vi "Lesson 3 - Exercise 3.1.1 - Complex Relationship Equations.vi"() -> ()   [LabVIEW 2016]
uses:
  <vilib>/Analysis/NI_AALBase.lvlib
panel:
  in  "Phase, deg":i32=30 step=15
  in  "Amplitude":i32=6 step=15
  out "A*Cos(f+phase)":dbl[](graph)=[5.196152422706632, 4.997527444260597, 4.779179508145178, 4.541970333910539, 4.286836077796821, 4.01478363815315, 3.7268866816698627, 3.4242814061065916, 3.1081620562387817, 2.779776210719172, 2.440419858454802, 2.091432283930893, 1.7341907816668303, 1.3701052206639366, 1.0006124802966145, 0.627170779605923, 0.25125392237519883, -0.12565451930013938, -0.5020670599938918, -0.8764981713744672, -1.2474701449065546, -1.6135189236915917, -1.973199880431498, -2.3250935187126154, -2.6678110751095634, -2.9999999999999973, -3.320349295460063, -3.6275946891742468, -3.920523623940631, -4.19798004308019, -4.458868952864364, -4.702160743955037, -4.926895254802223, -5.1321855609630385, -5.317221475387287, -5.4812727458556045, -5.623691936951348, -5.743916985192403, -5.84147341723896, -5.915976222423029, -5.967131372209639, -5.99473698059315, -5.998684100849072, -5.978957155497026, -5.93563399777793, -5.868885604402834, -5.778975400785949, -5.666258221424887, -5.531178909531004, -5.374270561436479, -5.196152422706633, -4.997527444260599, -4.779179508145179, -4.541970333910541, -4.286836077796822, -4.014783638153152, -3.7268866816698645, -3.4242814061065934, -3.1081620562387835, -2.7797762107191737, -2.4404198584548036, -2.091432283930895, -1.734190781666832, -1.3701052206639384, -1.0006124802966163, -0.6271707796059248, -0.2512539223752006, 0.1256545193001377, 0.50206705999389, 0.8764981713744657, 1.247470144906553, 1.6135189236915903, 1.9731998804314965, 2.325093518712614, 2.667811075109562, 2.9999999999999964, 3.320349295460062, 3.627594689174246, 3.92052362394063, 4.1979800430801895, 4.458868952864363, 4.702160743955036, 4.926895254802222, 5.132185560963038, 5.317221475387287, 5.481272745855604, 5.623691936951348, 5.743916985192403, 5.84147341723896, 5.915976222423029, 5.967131372209639, 5.99473698059315, 5.998684100849073, 5.978957155497027, 5.935633997777931, 5.868885604402836, 5.77897540078595, 5.666258221424889, 5.531178909531005, 5.3742705614364805]
  in  "I":dbl=5.196152422706632 format="%#.2g"
  in  "Q":dbl=2.9999999999999996 format="%#.2g"
  in  "stop":bool
  out "Q * Sin(f)":dbl[](graph)=[0.0, 0.18837155858794008, 0.3759997006929127, 0.5621439437571738, 0.7460696614945643, 0.9270509831248421, 1.1043736580540338, 1.2773378746952178, 1.4452610223051456, 1.6074803849369896, 1.7633557568774192, 1.9122719692460688, 2.0536413177860657, 2.186905882264234, 2.3115397283273675, 2.4270509831248415, 2.532983776506045, 2.62892004013159, 2.7144811573980583, 2.7893294576647536, 2.8531695488854605, 2.905749483385893, 2.9468617521860656, 2.976344103943433, 2.9940801852848145, 2.9999999999999996, 2.9940801852848145, 2.976344103943433, 2.9468617521860656, 2.905749483385893, 2.8531695488854605, 2.7893294576647536, 2.7144811573980583, 2.62892004013159, 2.532983776506045, 2.4270509831248415, 2.3115397283273675, 2.186905882264234, 2.0536413177860657, 1.9122719692460686, 1.7633557568774192, 1.6074803849369894, 1.4452610223051456, 1.2773378746952175, 1.1043736580540338, 0.9270509831248419, 0.7460696614945643, 0.5621439437571736, 0.3759997006929128, 0.18837155858793986, 5.551115123125783e-17, -0.1883715585879403, -0.37599970069291266, -0.562143943757174, -0.7460696614945642, -0.9270509831248424, -1.1043736580540338, -1.277337874695218, -1.4452610223051456, -1.6074803849369899, -1.7633557568774192, -1.912271969246069, -2.0536413177860657, -2.1869058822642344, -2.3115397283273675, -2.427050983124842, -2.532983776506045, -2.6289200401315904, -2.7144811573980583, -2.7893294576647536, -2.8531695488854605, -2.905749483385893, -2.9468617521860656, -2.976344103943433, -2.9940801852848145, -2.9999999999999996, -2.9940801852848145, -2.976344103943433, -2.9468617521860656, -2.905749483385893, -2.8531695488854605, -2.7893294576647536, -2.7144811573980583, -2.62892004013159, -2.532983776506045, -2.4270509831248415, -2.3115397283273675, -2.186905882264234, -2.0536413177860657, -1.9122719692460686, -1.7633557568774192, -1.6074803849369894, -1.4452610223051456, -1.2773378746952175, -1.1043736580540338, -0.9270509831248419, -0.7460696614945643, -0.5621439437571736, -0.3759997006929128, -0.18837155858793986]
  out "I * Cos(f)":dbl[](graph)=[5.196152422706632, 5.185899002848537, 5.15517920883809, 5.104114277667713, 5.032905739291384, 4.941834621277992, 4.831260339723896, 4.7016192808018085, 4.5534230785439265, 4.387256595656161, 4.20377561533222, 4.003704253176961, 3.787832099452895, 3.5570111029281697, 3.312152208623981, 3.054221762730764, 2.7842376988812427, 2.50326552083145, 2.2124140974041655, 1.9128312862902854, 1.6056994039789045, 1.2922305596943, 0.9736618717545665, 0.6512505852308165, 0.32626911017524973, 7.771561172376096e-16, -0.32626911017524984, -0.6512505852308149, -0.9736618717545666, -1.2922305596942985, -1.6056994039789045, -1.9128312862902839, -2.2124140974041655, -2.5032655208314485, -2.7842376988812427, -3.0542217627307626, -3.312152208623981, -3.5570111029281684, -3.787832099452895, -4.00370425317696, -4.20377561533222, -4.38725659565616, -4.5534230785439265, -4.701619280801808, -4.831260339723896, -4.941834621277991, -5.032905739291384, -5.104114277667712, -5.15517920883809, -5.1858990028485366, -5.196152422706632, -5.1858990028485366, -5.15517920883809, -5.104114277667712, -5.032905739291384, -4.941834621277991, -4.831260339723896, -4.701619280801808, -4.5534230785439265, -4.38725659565616, -4.20377561533222, -4.00370425317696, -3.787832099452895, -3.5570111029281692, -3.312152208623981, -3.0542217627307635, -2.7842376988812427, -2.50326552083145, -2.2124140974041655, -1.9128312862902854, -1.6056994039789045, -1.2922305596943002, -0.9736618717545665, -0.6512505852308169, -0.32626911017524973, -1.4432899320127035e-15, 0.32626911017524984, 0.651250585230814, 0.9736618717545666, 1.2922305596942973, 1.6056994039789045, 1.9128312862902825, 2.2124140974041655, 2.5032655208314467, 2.7842376988812427, 3.0542217627307604, 3.312152208623981, 3.557011102928166, 3.787832099452895, 4.0037042531769576, 4.20377561533222, 4.387256595656157, 4.5534230785439265, 4.701619280801805, 4.831260339723896, 4.941834621277988, 5.032905739291384, 5.104114277667709, 5.15517920883809, 5.185899002848534]
  out "I*Cos(f) - Q*Sin(f)":dbl[](graph)=[5.196152422706632, 4.997527444260597, 4.779179508145178, 4.541970333910539, 4.28683607779682, 4.014783638153149, 3.726886681669862, 3.4242814061065907, 3.108162056238781, 2.779776210719171, 2.440419858454801, 2.0914322839308923, 1.7341907816668294, 1.3701052206639357, 1.0006124802966134, 0.6271707796059225, 0.2512539223751977, -0.12565451930014016, -0.5020670599938928, -0.8764981713744682, -1.247470144906556, -1.6135189236915928, -1.973199880431499, -2.3250935187126167, -2.6678110751095647, -2.9999999999999987, -3.320349295460064, -3.627594689174248, -3.9205236239406323, -4.197980043080191, -4.458868952864365, -4.702160743955037, -4.926895254802224, -5.1321855609630385, -5.317221475387288, -5.481272745855604, -5.6236919369513485, -5.743916985192403, -5.84147341723896, -5.915976222423029, -5.967131372209639, -5.994736980593149, -5.998684100849072, -5.978957155497025, -5.935633997777929, -5.868885604402832, -5.778975400785948, -5.6662582214248856, -5.531178909531003, -5.374270561436476, -5.196152422706632, -4.997527444260596, -4.779179508145178, -4.5419703339105375, -4.28683607779682, -4.0147836381531485, -3.726886681669862, -3.42428140610659, -3.108162056238781, -2.77977621071917, -2.440419858454801, -2.0914322839308914, -1.7341907816668294, -1.3701052206639348, -1.0006124802966134, -0.6271707796059216, -0.2512539223751977, 0.1256545193001406, 0.5020670599938928, 0.8764981713744682, 1.247470144906556, 1.6135189236915926, 1.973199880431499, 2.3250935187126163, 2.6678110751095647, 2.9999999999999982, 3.320349295460064, 3.627594689174247, 3.9205236239406323, 4.19798004308019, 4.458868952864365, 4.702160743955036, 4.926895254802224, 5.132185560963037, 5.317221475387288, 5.481272745855602, 5.6236919369513485, 5.7439169851924, 5.84147341723896, 5.915976222423026, 5.967131372209639, 5.994736980593147, 5.998684100849072, 5.978957155497023, 5.935633997777929, 5.868885604402831, 5.778975400785948, 5.666258221424883, 5.531178909531003, 5.374270561436473]
  # "Run the program.\nCreate a signal by controlling the Phase (at the top).\nNotice how the amplitudes of two individual signals below are manipulated such that when combined, they also create the original signal."
  # "How does this work?"
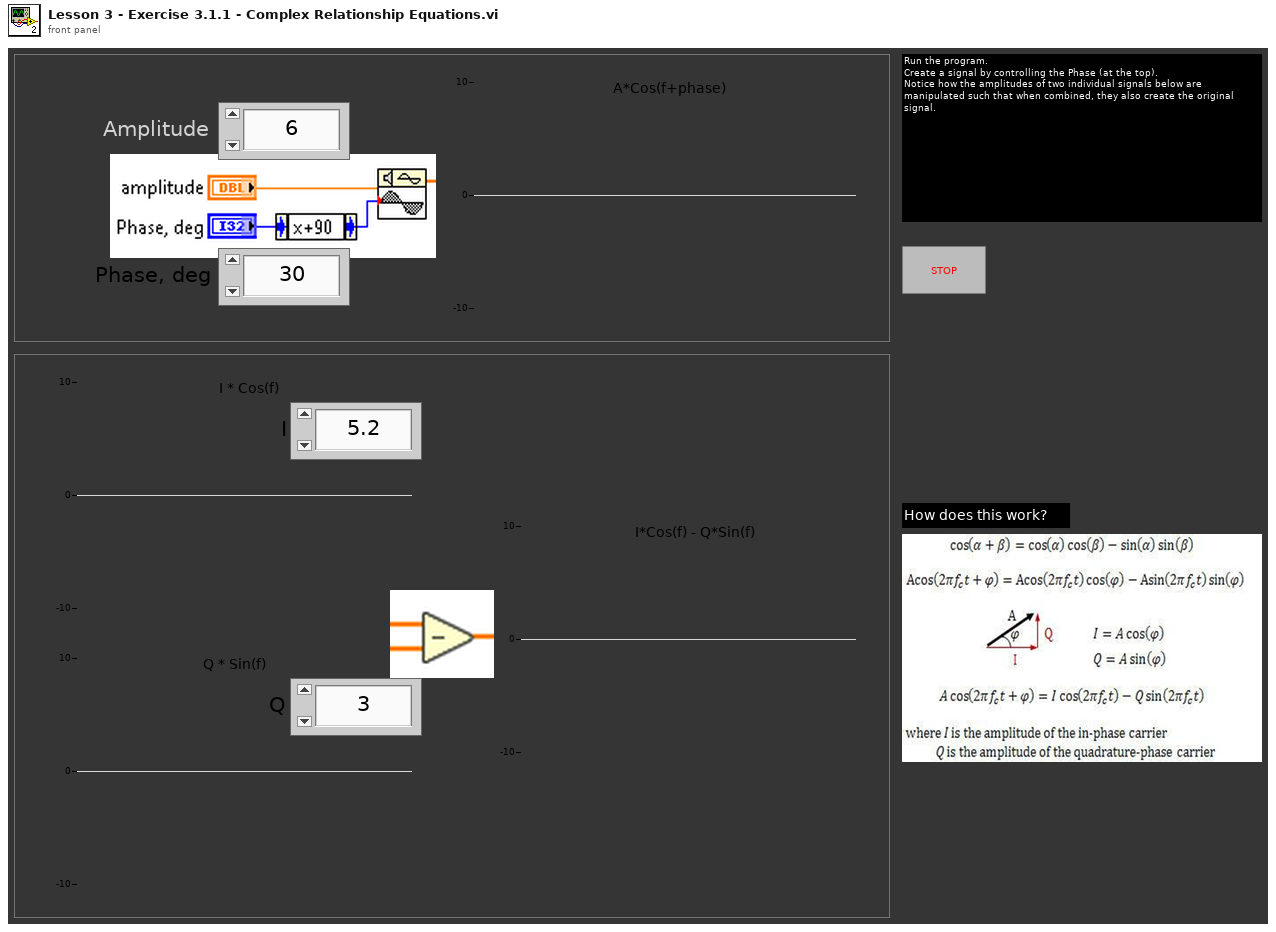
[diagram p1: front panel]
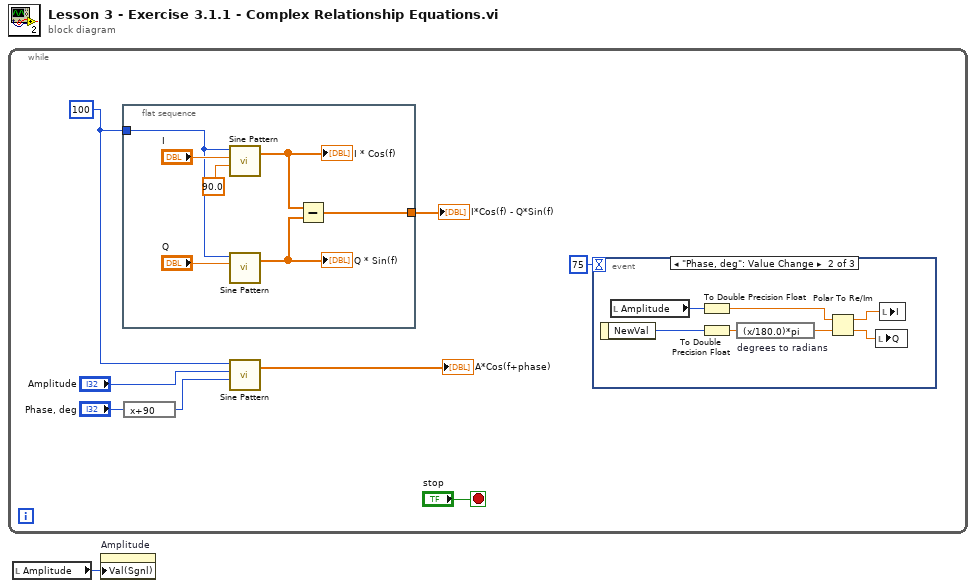
[diagram p0: block diagram]
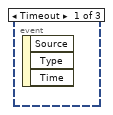
[diagram p2: hidden frame]
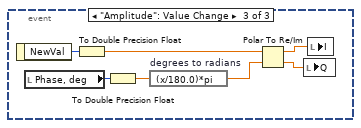
[diagram p3: hidden frame]
diagram:
  n1 = while {
    stop <- "stop" stop-if-true
    w2 = 100 ("samples")
    n2 = flat-sequence {
      tunnel: [w26] -> w9
      tunnel: w2 -> [w25]
      frame #0 {
        n3 = call <vilib>:"Sine Pattern.vi"("phase(degrees)"=90.0, "amplitude"="I", "samples"=w25) -> ("Sinusoidal Pattern"=w28:dbl[])  [unwired: 1 in, 1 out]
        "I * Cos(f)" <- w28
        n4 = call <vilib>:"Sine Pattern.vi"("amplitude"="Q", "samples"=w25) -> ("Sinusoidal Pattern"=w27:dbl[])  [unwired: 2 in, 1 out]
        "Q * Sin(f)" <- w27
        n5 = Subtract(x=w28, y=w27) -> (x-y=w26:dbl[])
      }
    }
    n6 = expression code="x+90"("Phase, deg") -> (w4:i32)
    n7 = call <vilib>:"Sine Pattern.vi"("phase(degrees)"=w4, "amplitude"="Amplitude", "samples"=w2) -> ("Sinusoidal Pattern"=→"A*Cos(f+phase)":dbl[])  [unwired: 1 in, 1 out]
    n8 = event shown="[1] \"Phase, deg\": Value Change" {
      selector: _ -> [_ _ _]
      dyn-events: _ -> [_ _ _]
      timeout: 75 -> [_ _ _]
      event Timeout {
        n9 = event-data() -> ()  [unwired: 1 in, 3 out]
      }
      event "Phase, deg": Value Change {
        n10 = event-data() -> ("NewVal"=w16:i32)  [unwired: 1 in]
        n11 = local read "Amplitude"() -> (w11:i32)
        n12 = To Double Precision Float(number=w11) -> (double precision float=w10:dbl)
        n13 = To Double Precision Float(number=w16) -> (double precision float=w14:dbl)
        n14 = expression code="(x/180.0)*pi" "degrees to radians"(w14) -> (w15:dbl)
        n15 = Polar To Re/Im(2:w15, 3:w10) -> (0:w12:dbl, 1:w13:dbl)
        n16 = local write "Q"(w12) -> ()
        n17 = local write "I"(w13) -> ()
      }
      event "Amplitude": Value Change {
        n18 = event-data() -> ("NewVal"=w23:i32)  [unwired: 1 in]
        n19 = local read "Phase, deg"() -> (w18:i32)
        n20 = To Double Precision Float(number=w23) -> (double precision float=w19:dbl)
        n21 = To Double Precision Float(number=w18) -> (double precision float=w17:dbl)
        n22 = expression code="(x/180.0)*pi" "degrees to radians"(w17) -> (w22:dbl)
        n23 = Polar To Re/Im(2:w22, 3:w19) -> (0:w20:dbl, 1:w21:dbl)
        n24 = local write "Q"(w20) -> ()
        n25 = local write "I"(w21) -> ()
      }
    }
    "I*Cos(f) - Q*Sin(f)" <- w9
  }
  n26 = local read "Amplitude"() -> (w1:i32)
  n27 = property on="Amplitude" class="DigNum (strict)"("Val(Sgnl)"=w1) -> ()  [unwired: 2 in, 2 out]
